vi "Msg Execute.vi"(10 "Msg":refnum<class "Msg.lvclass">, 11 "Base Actor in":refnum<class "Base Actor.lvclass">) -> (3 "Base Actor out":refnum<class "Base Actor.lvclass">)   [LabVIEW 2020, in "jettl.lvlib" / "Actor.lvlib" / "Base Actor.lvclass"]
uses:
  Base Actor.lvclass
  C:/git/jettl/src/jettl/jettl/Actor/Actor/Actor.lvclass
  Msg/Msg.lvclass
  Base Actor.lvclass/Base Actor.ctl
  Actor.lvlib
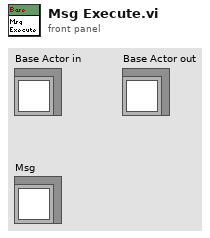
[diagram p1: front panel]
types:
  T1 = typedef "jettl.lvlib/Actor.lvlib/Msg Set.ctl" = set{refnum<class "Msg.lvclass">}
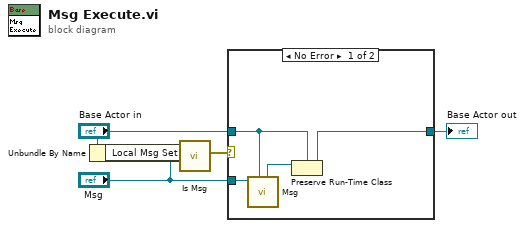
[diagram p0: block diagram]
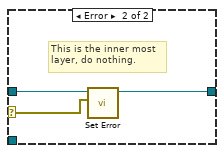
[diagram p2: hidden frame]
diagram:
  n1 = Unbundle By Name("Base Actor in") -> ("Local Msg Set"=w5:T1)
  n2 = call "Is Msg.vi"("Msg"="Msg", "Msgs"=w5) -> ("Error"=w4:errorcluster)  [unwired: 9 in]
  n3 = case shown="No Error" w4 {
    selector: w4 -> [_ w10]
    tunnel: "Base Actor in" -> [w7 w12]
    tunnel: [w6 w11] -> w2
    tunnel: "Msg" -> [w9 _]
    frame No Error {
      n4 = call-dynamic "Msg.vi"("Actor in"=w7, "Msg in"=w9) -> ("Actor out"=w8:refnum<class "Actor.lvclass">)  [unwired: 8 in, 1 out]
      n5 = Preserve Run-Time Class(object in=w8, 2:w7) -> (object out=w6:refnum<class "Base Actor.lvclass">)  [unwired: 1 in, 1 out]
    }
    frame Error {
      # "This is the inner most layer, do nothing."
      n6 = call-dynamic "Set Error.vi"("Error"=w10, "Base Actor in"=w12) -> ("Base Actor out"=w11:refnum<class "Base Actor.lvclass">)  [unwired: 9 in]
    }
  }
  "Base Actor out" <- w2
